vi "PAM Acquire Other Data TCP.vi"(1 "Other Data ID":refnum<k5>, 2 "icListen #":i32) -> (0 "Error Out":errorcluster)   [LabVIEW 2020]
uses:
  icListen 1 Synchronization.vi
  icListen 2 Synchronization.vi
  icListen 3 Synchronization.vi
  icListen 4 Synchronization.vi
  PAM Library.lvlib
panel:
  in  "Error In":errorcluster {"code" format="%.0x"}
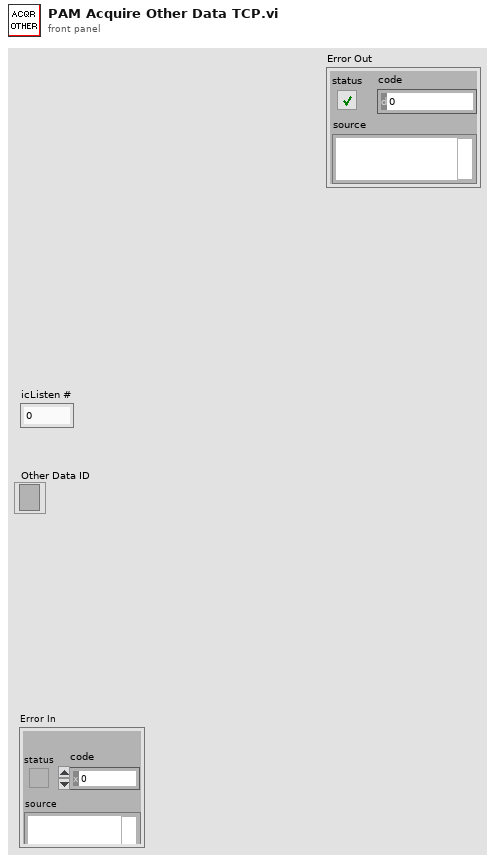
[diagram p1: front panel]
types:
  T1 = cluster{"System Time Status":u8, "Sync Status":u8, "PPS Count":u32, "Sync Offset":u32}
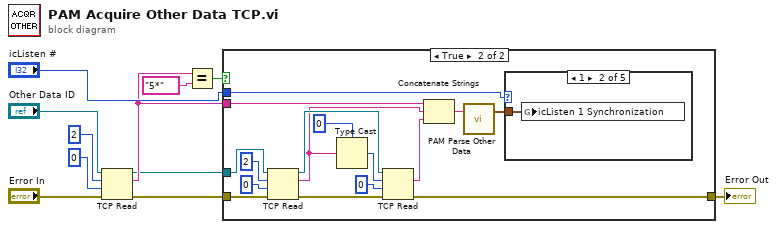
[diagram p0: block diagram]
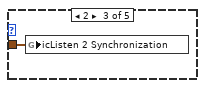
[diagram p4: hidden frame]
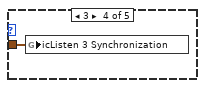
[diagram p5: hidden frame]
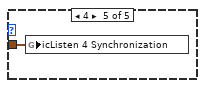
[diagram p6: hidden frame]
diagram:
  n1 = TCP Read(connection ID="Other Data ID", bytes to read=2 ("byte count"), error in (no error)="Error In", 9:0 ("timeout ms (25000)")) -> (connection ID out=w3:refnum<k5>, data out=w4:string, error out=w5:errorcluster)  [unwired: 1 in]
  n2 = Equal?(x=w4, y="5*" ("x")) -> (x = y?=w7:bool)
  n3 = case shown="True" w7 {
    tunnel: w3 -> [_ w15]
    tunnel: w5 -> [w12 w27]
    tunnel: w4 -> [_ w22]
    tunnel: "icListen #" -> [_ w17]
    tunnel: [w12 w18] -> w1
    frame False {
    }
    frame True {
      n4 = TCP Read(connection ID=w15, bytes to read=2 ("byte count"), error in (no error)=w27, 9:0 ("timeout ms (25000)")) -> (connection ID out=w24:refnum<k5>, data out=w21:string, error out=w23:errorcluster)  [unwired: 1 in]
      n5 = Type Cast(type=0, x=w21) -> (*(type *) &x=w25:i32)
      n6 = TCP Read(connection ID=w24, bytes to read=w25, error in (no error)=w23, 9:0 ("timeout ms (25000)")) -> (data out=w20:string, error out=w18:errorcluster)  [unwired: 1 in, 1 out]
      n7 = Concatenate Strings(w22, w21, w20) -> (w19:string)
      n8 = call "PAM Parse Other Data.vi"("Header"=w19) -> ("Synchronization"=w16:T1)  [unwired: 16 in, 2 out]
      n9 = case shown="1" w17 {
        tunnel: w16 -> [_ w29 w30 w31 w32]
        frame 0, Default {
        }
        frame 1 {
          n10 = global write "icListen 1 Synchronization.vi" "icListen 1 Synchronization"(w29) -> ()
        }
        frame 2 {
          n11 = global write "icListen 2 Synchronization.vi" "icListen 2 Synchronization"(w30) -> ()
        }
        frame 3 {
          n12 = global write "icListen 3 Synchronization.vi" "icListen 3 Synchronization"(w31) -> ()
        }
        frame 4 {
          n13 = global write "icListen 4 Synchronization.vi" "icListen 4 Synchronization"(w32) -> ()
        }
      }
    }
  }
  "Error Out" <- w1
